vi "SUB_RTXDll_Write.vi"(1 "CMD":string="*IDN?") -> ()   [LabVIEW 2011]
uses:
  R2012dll.dll
panel:
  out "error out":errorcluster
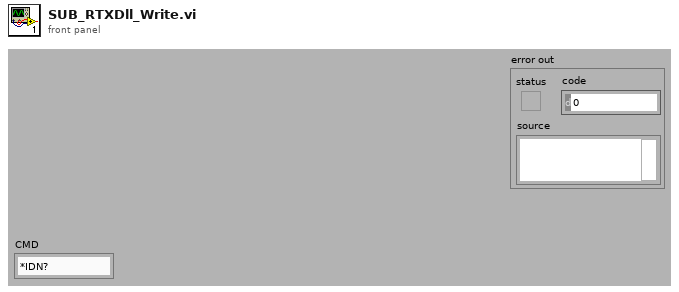
[diagram p1: front panel]
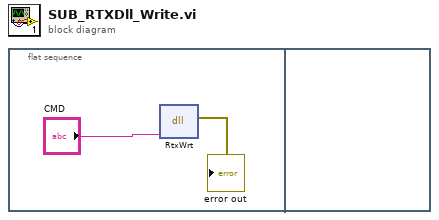
[diagram p0: block diagram]
diagram:
  n1 = flat-sequence {
    frame #0 {
      n2 = dll-call lib="E:/Konftel_Project/R2012dll.dll" fn="RtxWrt"("RtxWrt"="CMD") -> (error out=→"error out":errorcluster)  [unwired: 5 in, 1 out]
    }
    frame #1 {
    }
  }
